vi "DriveToPoint.vi"() -> ()   [LabVIEW 2018]
uses:
  <vilib>/Studica/Studica Toolkit/Background/Mxp Selection.ctl
panel:
  in  "Linear Hoist":dbl(slide) scale=-1.0..1.0
  in  "StopMotors":bool
  in  "Robot Model":string(combo)="3-wheeled"
  in  "Stop Program 2":bool
  out "PID-Output":dbl[](array[numeric])=[0.004570312508683128, 0.004570312508683128, 0.004570312508683128, 0.004570312508683128]
  in  "Reset Encoders":bool
  out "Actual-SpeedList":dbl[](array[numeric])
  out "Tick Count(uSec)":u32=4696177 caption="Tick Count(Ticks)"
  out "Wheel Distances Travelled":dbl[](array[numeric])
  in  "Stop Program":bool
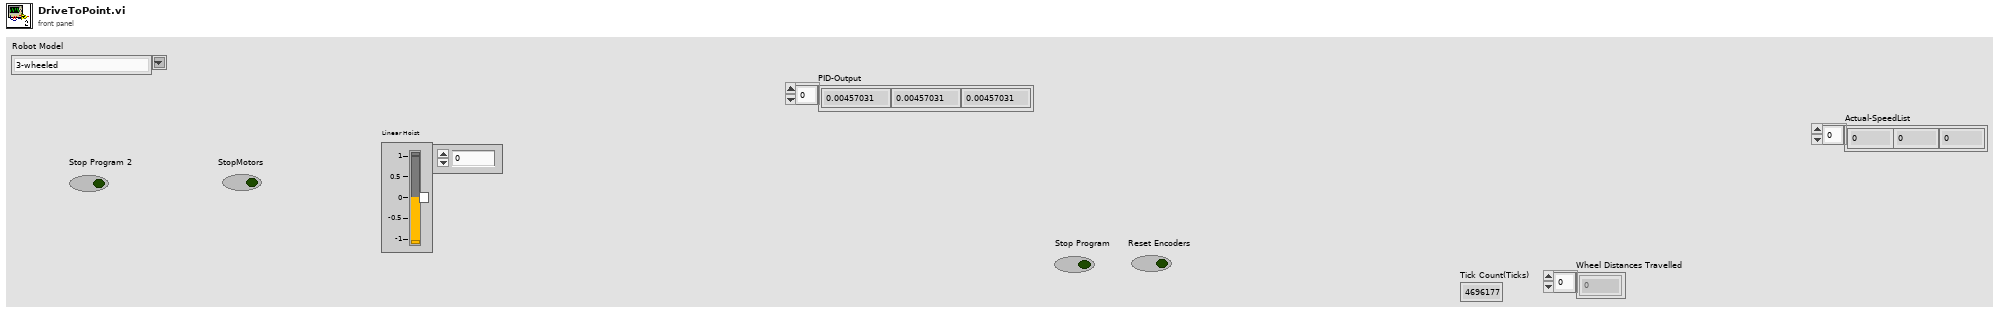
[diagram p1: front panel]
types:
  T1 = typedef "Mxp Selection.ctl" = enum16{"MXP A", "MXP B"}
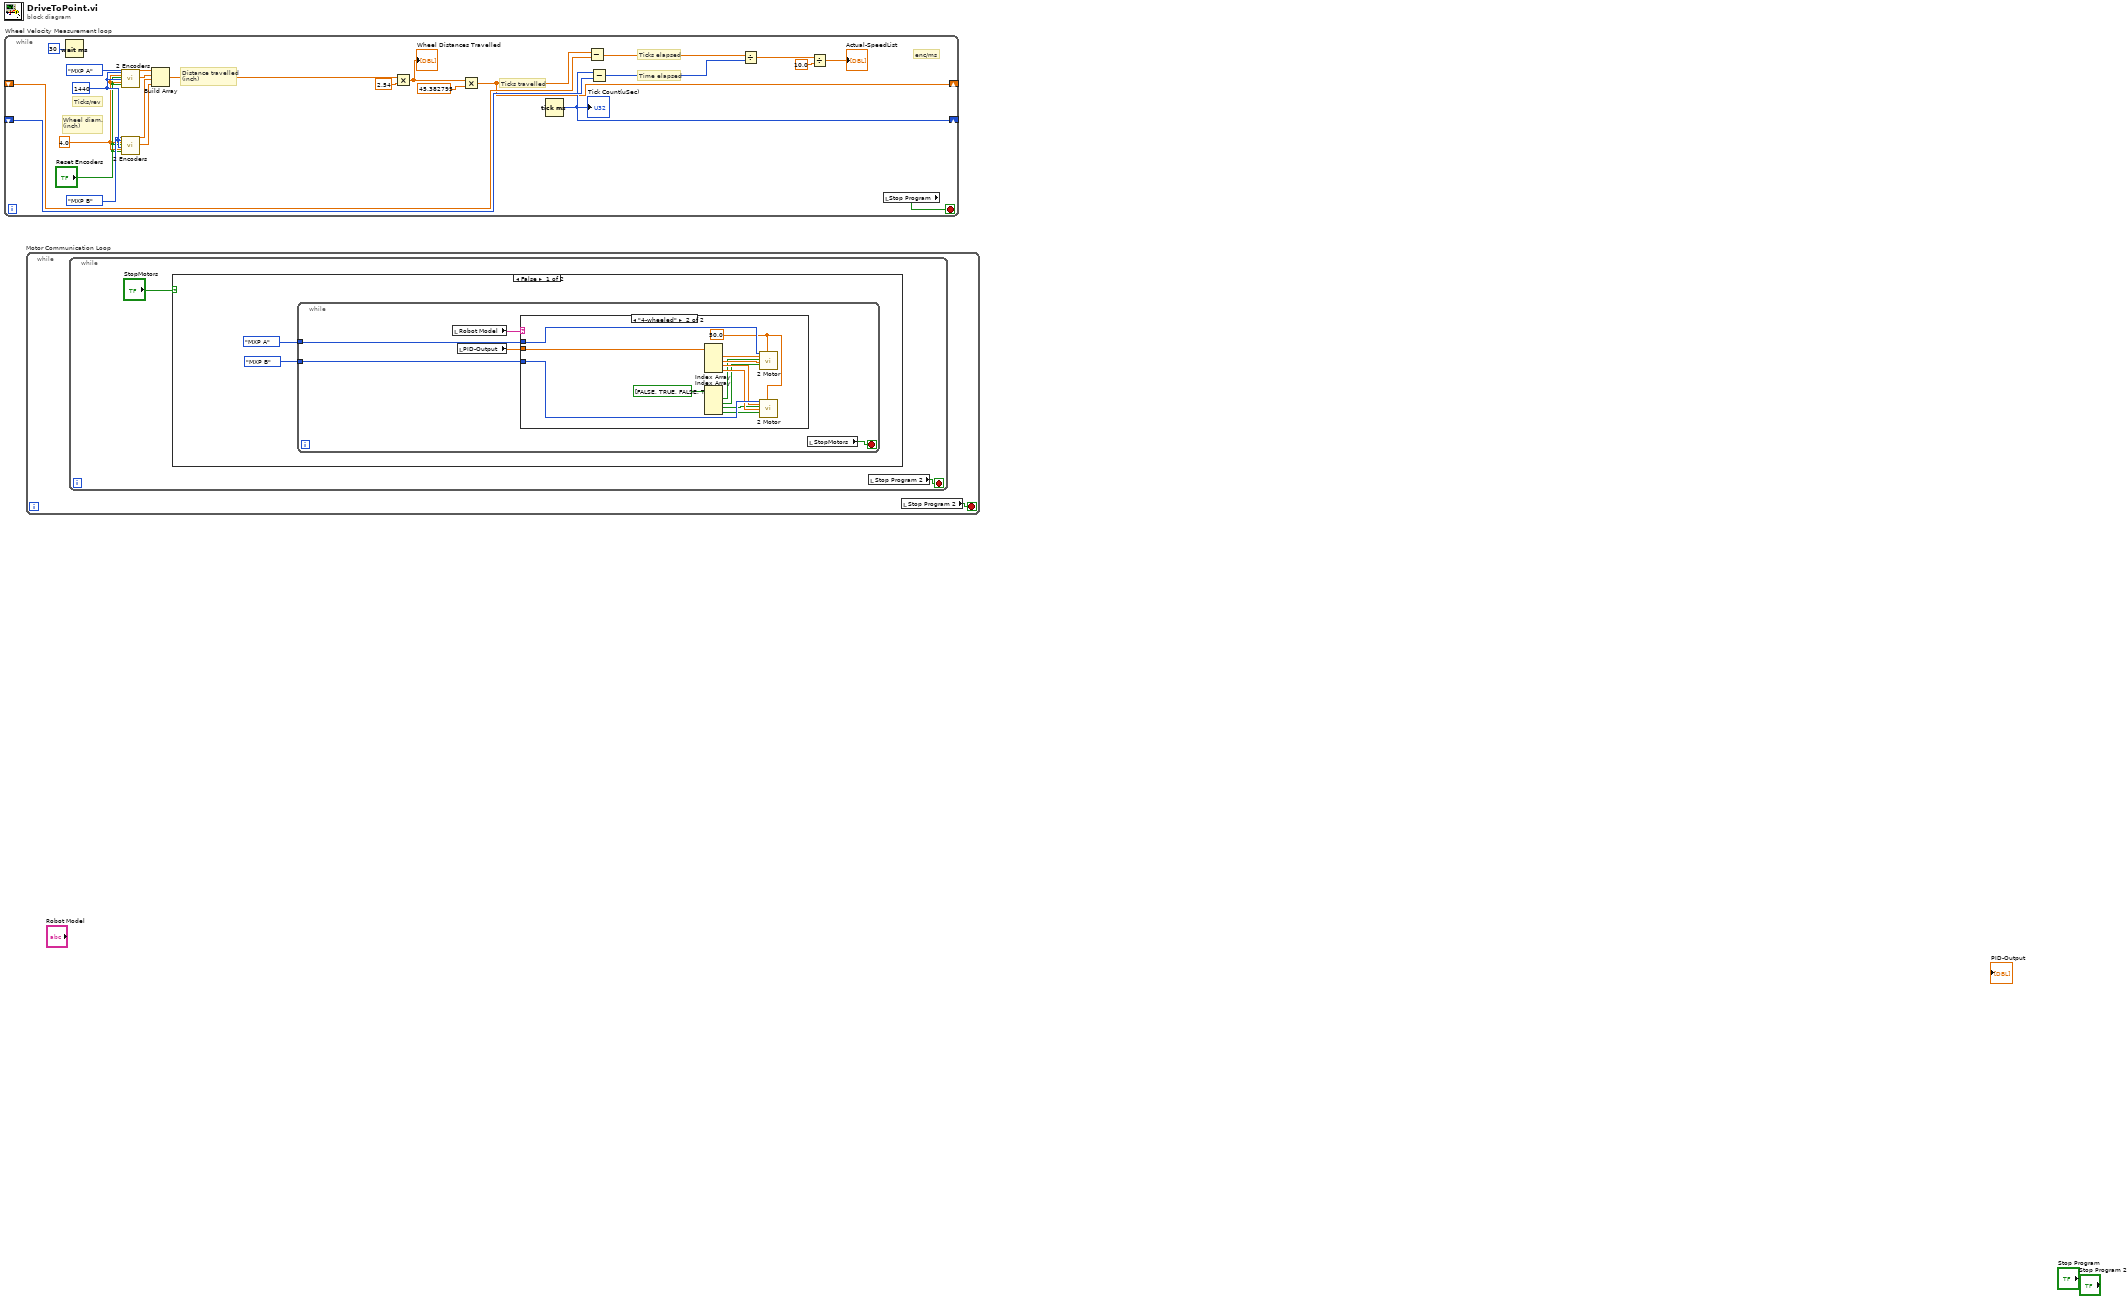
[diagram p0: block diagram]
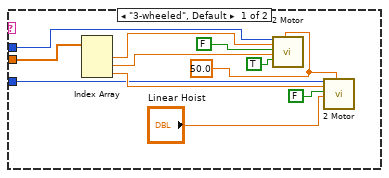
[diagram p2: hidden frame]
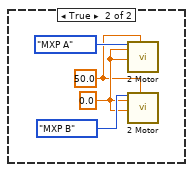
[diagram p3: hidden frame]
diagram:
  n1 = while "Wheel Velocity Measurement loop" {
    shift-right: [w9] -> _
    shift-left: _ -> [w14]
    shift-right: [w10] -> _
    shift-left: _ -> [w12]
    stop <- w2 stop-if-true
    w7 = 4.0 ("Wheel Diameter M1 (inches)")
    w17 = u32 1440 ("Ticks Per Rev M0")
    # "Ticks travelled"
    # "Distance travelled\n(inch)"
    # "Wheel diam.\n(inch)"
    # "Ticks/rev"
    # "Ticks elapsed"
    # "Time elapsed"
    # "enc/ms"
    n2 = Wait (ms)(milliseconds to wait=u32 30) -> ()  [unwired: 1 out]
    n3 = call <vilib>:"2 Encoders.vi"("Mxp Side"=Mxp_Selection."MXP A", "Ticks Per Rev M0"=w17, "Wheel Diameter M0 (inches)"=w7, "Reset Encoder 0"="Reset Encoders", "Ticks Per Rev M1"=w17, "Wheel Diameter M1 (inches)"=w7, "Reset Encoder 1"="Reset Encoders") -> ("Distance M0 (inches)"=w18:dbl, "Distance M1 (inches)"=w19:dbl)  [unwired: 18 in, 1 out]
    n4 = call <vilib>:"2 Encoders.vi"("Mxp Side"=Mxp_Selection."MXP B", "Ticks Per Rev M0"=w17, "Wheel Diameter M0 (inches)"=w7, "Reset Encoder 0"="Reset Encoders", "Ticks Per Rev M1"=w17, "Wheel Diameter M1 (inches)"=w7, "Reset Encoder 1"="Reset Encoders") -> ("Distance M0 (inches)"=w20:dbl, "Distance M1 (inches)"=w8:dbl)  [unwired: 18 in, 1 out]
    n5 = Build Array(w18, w19, w20, w8) -> (w22:dbl[])
    n6 = Multiply(x=w22, y=2.54) -> (x*y=w1:dbl[])
    "Wheel Distances Travelled" <- w1
    n7 = Multiply(x=w1, y=45.382795) -> (x*y=w9:dbl[])
    n8 = Tick Count (ms)() -> (millisecond timer value=w10:u32)
    "Tick Count(uSec)" <- w10
    n9 = Subtract(x=w9, y=w14) -> (x-y=w13:dbl[])
    n10 = Subtract(x=w10, y=w12) -> (x-y=w24:u32)
    n11 = Divide(x=w13, y=w24) -> (x/y=w5:dbl[])
    n12 = Divide(x=w5, y=10.0) -> (x/y=→"Actual-SpeedList":dbl[])
    n13 = local read "Stop Program"() -> (w2:bool)
  }
  n14 = while "Motor Communication Loop" {
    stop <- w25 stop-if-true
    n15 = while {
      stop <- w26 stop-if-true
      n16 = case shown="False" "StopMotors" {
        frame False {
          n17 = while {
            tunnel: Mxp_Selection."MXP A" ("Mxp Side") -> [w34]
            tunnel: Mxp_Selection."MXP B" ("Mxp Side") -> [w33]
            stop <- w30 stop-if-true
            n18 = local read "Robot Model"() -> (w32:string)
            n19 = local read "PID-Output"() -> (w31:dbl[])
            n20 = case shown="\"4-wheeled\"" w32 {
              tunnel: w34 -> [w37 w58]
              tunnel: w33 -> [w36 w57]
              tunnel: w31 -> [w38 w46]
              frame "3-wheeled", Default {
                w45 = 50.0 ("Frequency [Hz]")
                n21 = Index Array(array=w38) -> (element #1=w41:dbl, element #2=w40:dbl, element #3=w39:dbl)  [unwired: 3 in]
                n22 = call <vilib>:"2 Motor.vi"("Mxp Side"=w37, "Speed M0"=w41, "Invert M0"=FALSE, "Speed M1"=w40, "Invert M1"=TRUE ("Invert M0"), "Frequency [Hz]"=w45) -> ()  [unwired: 13 in, 1 out]
                n23 = call <vilib>:"2 Motor.vi"("Mxp Side"=w36, "Speed M0"=w39, "Invert M0"=FALSE, "Speed M1"="Linear Hoist", "Frequency [Hz]"=w45) -> ()  [unwired: 14 in, 1 out]
              }
              frame "4-wheeled" {
                w56 = 50.0 ("Frequency [Hz]")
                n24 = Index Array(array=w46) -> (element #1=w55:dbl, element #2=w54:dbl, element #3=w53:dbl, element #4=w52:dbl)  [unwired: 4 in]
                n25 = Index Array(array=bool[] [FALSE, TRUE, FALSE, TRUE] ("Motor Directions")) -> (element #1=w50:bool, element #2=w49:bool, element #3=w48:bool, element #4=w47:bool)  [unwired: 4 in]
                n26 = call <vilib>:"2 Motor.vi"("Mxp Side"=w58, "Speed M0"=w55, "Invert M0"=w50, "Speed M1"=w54, "Invert M1"=w49, "Frequency [Hz]"=w56) -> ()  [unwired: 13 in, 1 out]
                n27 = call <vilib>:"2 Motor.vi"("Mxp Side"=w57, "Speed M0"=w53, "Invert M0"=w48, "Speed M1"=w52, "Invert M1"=w47, "Frequency [Hz]"=w56) -> ()  [unwired: 13 in, 1 out]
              }
            }
            n28 = local read "StopMotors"() -> (w30:bool)
          }
        }
        frame True {
          w59 = 50.0 ("Frequency [Hz]")
          w60 = 0.0 ("Speed M0")
          n29 = call <vilib>:"2 Motor.vi"("Mxp Side"=Mxp_Selection."MXP A", "Speed M0"=w60, "Speed M1"=w60, "Frequency [Hz]"=w59) -> ()  [unwired: 15 in, 1 out]
          n30 = call <vilib>:"2 Motor.vi"("Mxp Side"=Mxp_Selection."MXP B", "Speed M0"=w60, "Speed M1"=w60, "Frequency [Hz]"=w59) -> ()  [unwired: 15 in, 1 out]
        }
      }
      n31 = local read "Stop Program 2"() -> (w26:bool)
    }
    n32 = local read "Stop Program 2"() -> (w25:bool)
  }
